vi "Initialize Library.vi"(8 "error in (no error)":errorcluster) -> (0 "error out":errorcluster, 2 "KHEL Event":refnum<user-event>)   [LabVIEW 2016, in "Hall Effect Library.lvlib"]
doc: "This VI initializes the Keithley Hall Effect Library, readying it for use. This VI should be called before any other VI in the library.\n\n<b>Event Queue Ref In</b> is a reference to your main application's event queue. It allows the library to send events to your application."
uses:
  Hall Effect Library.lvlib
  Controls/Message Types.ctl
  Private/Global Variables/Communication.vi
  Private/Global Variables/Hall Effect Data.vi
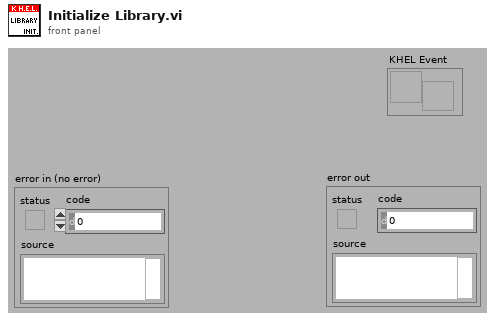
[diagram p1: front panel]
types:
  T1 = typedef "Hall Effect Library.lvlib/Message Types.ctl" = enum16{"Status", "New Data", "Test End Normal", "Test End User Abort", "Test End Error"}
  T2 = cluster{"RAvg":dbl, "RH1":dbl, "RH2":dbl, "uH":dbl}
  T3 = cluster{"RHD":dbl, "RHC":dbl, "RHAvg":dbl, "uH":dbl, "n/p":dbl}
  T4 = cluster{"fA":dbl, "fB":dbl, "QA":dbl, "QB":dbl, "pAvg":dbl, "pA":dbl, "pB":dbl}
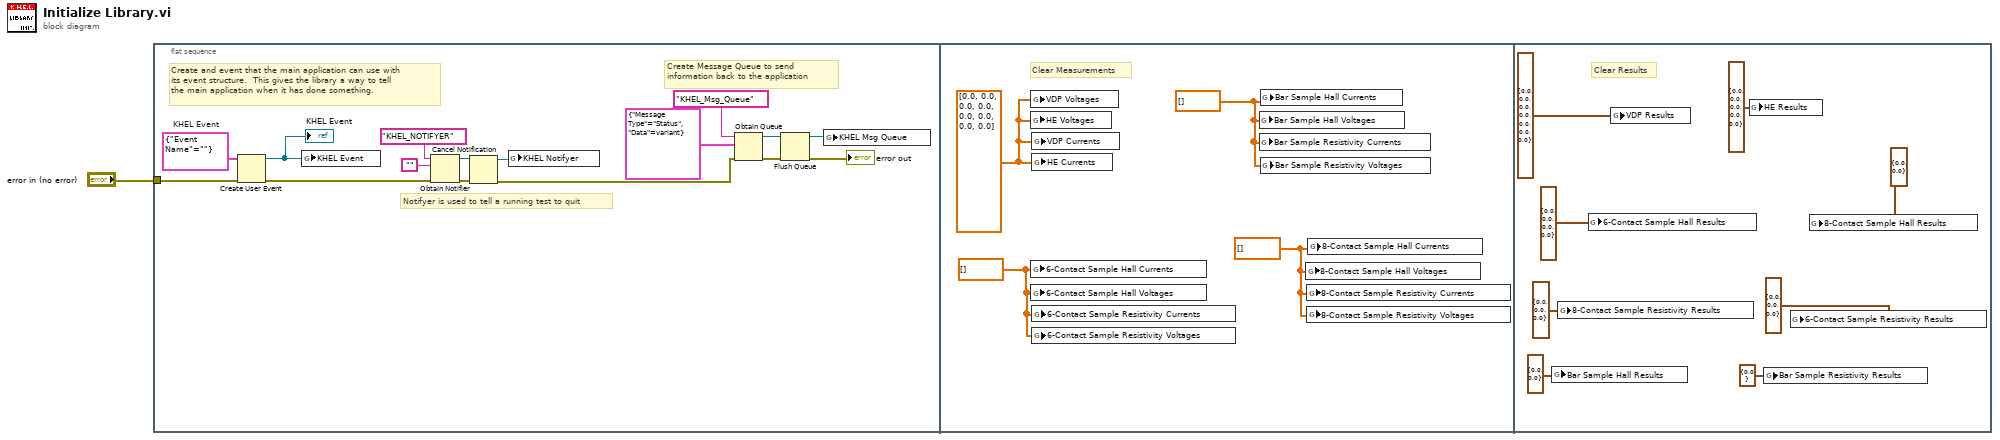
[diagram p0: block diagram]
diagram:
  n1 = flat-sequence {
    tunnel: "error in (no error)" -> [w4]
    frame #0 {
      w3 = cluster{"Event Name":string} {"Event Name"=""}  # KHEL Event
      # "Create and event that the main application can use with\nits event structure.  This gives the library a way to tell\nthe main application when it has done something."
      # "Notifyer is used to tell a running test to quit"
      # "Create Message Queue to send\ninformation back to the application"
      n2 = Create User Event(user event datatype=w3, error in=w4) -> (user event=w2:refnum<user-event>, error out=w5:errorcluster)
      "KHEL Event" <- w2
      n3 = global write "Communication.vi" "KHEL Event"(w2) -> ()
      n4 = Obtain Notifier(name (unnamed)="KHEL_NOTIFYER", notification data type="", error in (no error)=w5) -> (notifier out=w8:refnum<notifier>, error out=w7:errorcluster)  [unwired: 1 in, 1 out]
      n5 = Cancel Notification(0:w8, 3:w7) -> (8:w6:refnum<notifier>, 11:w15:errorcluster)  [unwired: 1 out]
      n6 = global write "Communication.vi" "KHEL Notifyer"(w6) -> ()
      n7 = Obtain Queue(name (unnamed)="KHEL_Msg_Queue", element data type=cluster{"Message Type":T1, "Data":variant} {"Message Type"=enum."Status", "Data"=variant}, error in (no error)=w15) -> (queue out=w13:refnum<queue>, error out=w14:errorcluster)  [unwired: 2 in, 1 out]
      n8 = Flush Queue(queue=w13, error in (no error)=w14) -> (queue out=w12:refnum<queue>, error out=→"error out":errorcluster)  [unwired: 1 out]
      n9 = global write "Communication.vi" "KHEL Msg Queue"(w12) -> ()
    }
    frame #1 {
      w18 = dbl[] [] ("8-Contact Sample Hall Currents")
      w19 = dbl[] [] ("6-Contact Sample Hall Currents")
      w20 = dbl[] [] ("Bar Sample Hall Currents")
      w21 = dbl[] [0.0, 0.0, 0.0, 0.0, 0.0, 0.0, 0.0, 0.0] ("Van Der Pauw Voltages")
      # "Clear Measurements"
      n10 = global write "Hall Effect Data.vi" "VDP Voltages"(w21) -> ()
      n11 = global write "Hall Effect Data.vi" "HE Voltages"(w21) -> ()
      n12 = global write "Hall Effect Data.vi" "6-Contact Sample Hall Currents"(w19) -> ()
      n13 = global write "Hall Effect Data.vi" "6-Contact Sample Hall Voltages"(w19) -> ()
      n14 = global write "Hall Effect Data.vi" "VDP Currents"(w21) -> ()
      n15 = global write "Hall Effect Data.vi" "HE Currents"(w21) -> ()
      n16 = global write "Hall Effect Data.vi" "6-Contact Sample Resistivity Currents"(w19) -> ()
      n17 = global write "Hall Effect Data.vi" "6-Contact Sample Resistivity Voltages"(w19) -> ()
      n18 = global write "Hall Effect Data.vi" "Bar Sample Hall Voltages"(w20) -> ()
      n19 = global write "Hall Effect Data.vi" "Bar Sample Resistivity Currents"(w20) -> ()
      n20 = global write "Hall Effect Data.vi" "Bar Sample Hall Currents"(w20) -> ()
      n21 = global write "Hall Effect Data.vi" "Bar Sample Resistivity Voltages"(w20) -> ()
      n22 = global write "Hall Effect Data.vi" "8-Contact Sample Hall Voltages"(w18) -> ()
      n23 = global write "Hall Effect Data.vi" "8-Contact Sample Resistivity Currents"(w18) -> ()
      n24 = global write "Hall Effect Data.vi" "8-Contact Sample Resistivity Voltages"(w18) -> ()
      n25 = global write "Hall Effect Data.vi" "8-Contact Sample Hall Currents"(w18) -> ()
    }
    frame #2 {
      # "Clear Results"
      n26 = global write "Hall Effect Data.vi" "Bar Sample Hall Results"(cluster{"n/p":dbl, "uH":dbl} {"n/p"=0.0, "uH"=0.0} ("Bar Sample Hall Results")) -> ()
      n27 = global write "Hall Effect Data.vi" "8-Contact Sample Resistivity Results"(cluster{"PAvg":dbl, "PA":dbl, "PB":dbl} {"PAvg"=0.0, "PA"=0.0, "PB"=0.0} ("8-Contact Sample Resistivity Results")) -> ()
      n28 = global write "Hall Effect Data.vi" "6-Contact Sample Hall Results"(T2 {"RAvg"=0.0, "RH1"=0.0, "RH2"=0.0, "uH"=0.0} ("6-Contact Sample Hall Results")) -> ()
      n29 = global write "Hall Effect Data.vi" "VDP Results"(T4 {"fA"=0.0, "fB"=0.0, "QA"=0.0, "QB"=0.0, "pAvg"=0.0, "pA"=0.0, "pB"=0.0} ("Van Der Pauw Results")) -> ()
      n30 = global write "Hall Effect Data.vi" "HE Results"(T3 {"RHD"=0.0, "RHC"=0.0, "RHAvg"=0.0, "uH"=0.0, "n/p"=0.0} ("HE Results")) -> ()
      n31 = global write "Hall Effect Data.vi" "Bar Sample Resistivity Results"(cluster{"p":dbl} {"p"=0.0} ("Bar Sample Resistivity Results")) -> ()
      n32 = global write "Hall Effect Data.vi" "6-Contact Sample Resistivity Results"(cluster{"PAvg":dbl, "PA":dbl, "PB":dbl} {"PAvg"=0.0, "PA"=0.0, "PB"=0.0} ("6-Contact Sample Resistivity Results")) -> ()
      n33 = global write "Hall Effect Data.vi" "8-Contact Sample Hall Results"(cluster{"RH":dbl, "uH":dbl} {"RH"=0.0, "uH"=0.0} ("8-Contact Sample Hall Results")) -> ()
    }
  }
